vi "NI VeriStand - Get Custom Device Runtime Configuration Ref.vi"(8 "error in":errorcluster, 11 "Runtime Configuration Ref":refnum<k24>) -> (0 "error out":errorcluster, 2 "Parent Ref":T1 format="%.0x", 3 "Runtime Configuration Ref out":refnum<k24>)   [LabVIEW 2025, in "NI_VS RuntimeConfigurationFile ScriptingAPI.lvlib"]
uses:
  NI_VS RuntimeConfigurationFile ScriptingAPI.lvlib
  <vilib>/NI VeriStand/Custom Device API/Custom Device API.lvlib
  NationalInstruments.VeriStand.SystemDefinitionAPI
  <vilib>/NI VeriStand/Custom Device API/Custom Device Item Ref.ctl
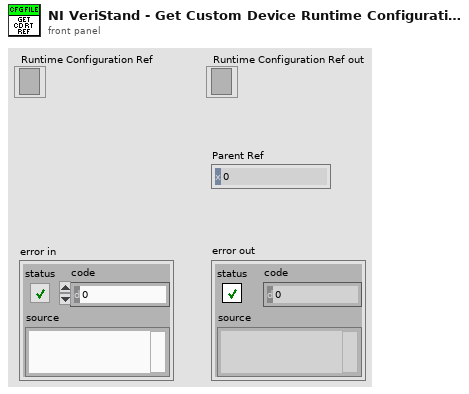
[diagram p1: front panel]
types:
  T1 = typedef "Custom Device API.lvlib/Custom Device Item Ref.ctl" = u64
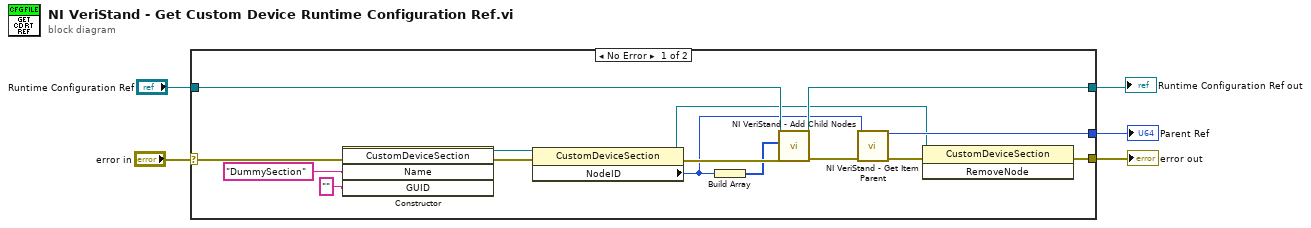
[diagram p0: block diagram]
diagram:
  n1 = case shown="No Error" "error in" {
    selector: "error in" -> [w16 w22]
    tunnel: "Runtime Configuration Ref" -> [w14 w21]
    tunnel: [w13 w21] -> w2
    tunnel: [w11 _] -> w1
    tunnel: [w18 w22] -> w5
    frame No Error {
      n2 = constructor class="CustomDeviceSection"(error in=w16, "Name"="DummySection", "GUID"="") -> (reference out=w10:refnum<k24>, error out=w17:errorcluster)  [unwired: 2 in, 3 out]
      n3 = property class="CustomDeviceSection"(reference=w10, error in=w17) -> (reference out=w9:refnum<k24>, error out=w15:errorcluster, "NodeID"=w8:u64)
      n4 = Build Array(w8) -> (w12:u64[])
      n5 = call "NI VeriStand - Add Child Nodes.vi"("Error in"=w15, "Child Nodes"=w12, "Runtime Configuration Ref in"=w14) -> ("Error out"=w20:errorcluster, "Runtime Configuration Ref out"=w13:refnum<k24>)  [unwired: 5 in, 2 out]
      n6 = call <vilib>:"NI VeriStand - Get Item Parent.vi"("error in (no error)"=w20, "Item Ref in"=w8) -> ("error out"=w19:errorcluster, "Parent Ref"=w11:T1)  [unwired: 6 in, 2 out]
      n7 = invoke class="CustomDeviceSection" method="RemoveNode"(reference=w9, error in=w19) -> (error out=w18:errorcluster)  [unwired: 1 in, 2 out]
    }
    frame Error {
    }
  }
  "Parent Ref" <- w1
  "error out" <- w5
  "Runtime Configuration Ref out" <- w2
